vi "MAIN FPGA.vi"() -> ()   [LabVIEW 2019]
uses:
  <vilib>/rvi/Emulation/niFpgaGetClockAttributes.vi
  <vilib>/rvi/Emulation/niFpgaSctlEmulationGetInTimedLoop.vi
  <vilib>/rvi/Emulation/niFpgaEmulationReportErrorSimple.vi
  <vilib>/rvi/eio/common/nirviEmuTemplateMethod_errors.vi
  <vilib>/rvi/Emulation/niFpgaCriticalErrorInLSC.vi
  <vilib>/eio/EIONode/EIONode.xnode
panel:
  out "AI1":fxp<+/-,21,-4>
  out "dt ticks":u32
  out "AI0":fxp<+/-,21,-4>
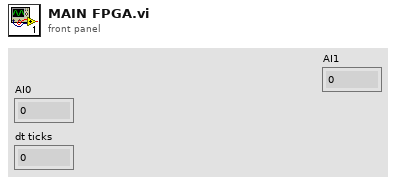
[diagram p1: front panel]
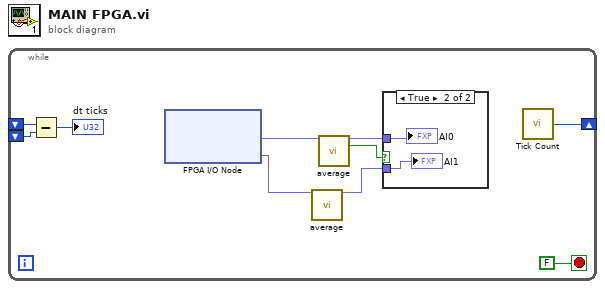
[diagram p0: block diagram]
diagram:
  n1 = while {
    shift-right: [w6] -> _
    shift-left: _ -> [w5]
    shift-left: _ -> [w4]
    stop <- FALSE stop-if-true
    n2 = Subtract(x=w5, y=w4) -> (x-y=→"dt ticks":u32)
    n3 = xnode "FPGA I/O Node"() -> ("Mod1/AI0"=w9:fxp<+/-,21,-4>, "Mod1/AI1"=w2:fxp<+/-,21,-4>)  [unwired: 2 in, 2 out]
    n4 = call "average.vi"("Mod1/AI0"=w2) -> ("mean"=w1:fxp<+/-,21,-4>)  [unwired: 13 in, 1 out]
    n5 = call "average.vi"("Mod1/AI0"=w9) -> ("mean"=w7:fxp<+/-,21,-4>, "output valid"=w8:bool)  [unwired: 13 in]
    n6 = case shown="True" w8 {
      tunnel: w7 -> [_ w12]
      tunnel: w1 -> [_ w11]
      frame False {
      }
      frame True {
        "AI0" <- w12
        "AI1" <- w11
      }
    }
    n7 = call "Tick Count"() -> ("Tick Count(Ticks)"=w6:u32)
  }
